vi "LJM read config.vi"(0 "Working Directory":path, 5 "filename":string="ljstreamud.cfg") -> (1 "Data File Prefix":string="data", 2 "Scan Rate (Hz)":dbl=500.0 format="%.3f", 3 "Graph History":i32=1000 min=0, 4 "# Channels":i32=4, 6 "Disable Scaling":bool, 8 "Max File Size (Bytes)":i32=1048576, 9 "Write To File":bool, 10 "Channel Setup":T1={"+Ch"=["0", "1", "2", "3", "4", "5", "6", "7"], "-Ch"=["199", "199", "199", "199", "199", "199", "199", "199"], "Ranges"=[0, 0, 0, 0, 0, 0, 0, 0], "Scaling Equation"=["y=v0", "y=v1", "y=v2", "y=v3", "y=v4", "y=v5", "y=v6", "y=v7"], "Graph?"=[]} {"Ranges" items=["LJ_rgBIP10V", "LJ_rgBIP5V", "LJ_rgUNI5V", "LJ_rgUNI2P5V", "LJ_rgUNI1P25V", "LJ_rgBIP1V", "LJ_rgUNIP625V", "LJ_rgBIPP1V", "LJ_rgBIPP01V"]}, 11 "Good Experiment Config":bool, 12 "Interval (ms)":u32=500, 13 "Resolution":u8, 14 "SettlingFactor":u8, 15 "error out":errorcluster)   [LabVIEW 2025]
uses:
  <vilib>/Utility/config.llb/Read Key (String).vi
  <vilib>/Utility/config.llb/Read Key (U32).vi
  <vilib>/Utility/config.llb/Read Key (Double).vi
  <vilib>/Utility/config.llb/Read Key (I32).vi
  <vilib>/Utility/config.llb/Read Key (Boolean).vi
  <vilib>/Utility/config.llb/NI_LVConfig.lvlib
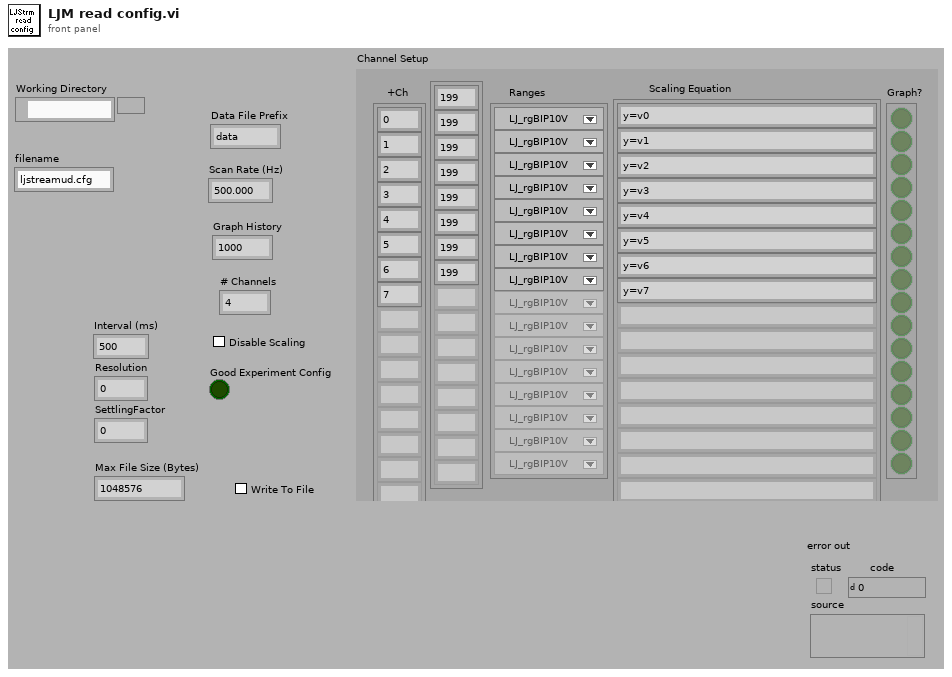
[diagram p1: front panel]
types:
  T1 = cluster{"+Ch":string[], "-Ch":string[], "Ranges":u16[], "Scaling Equation":string[], "Graph?":bool[]}
  T2 = typedef "NI_LVConfig.lvlib/Config Data RefNum.ctl" = refnum<k1>
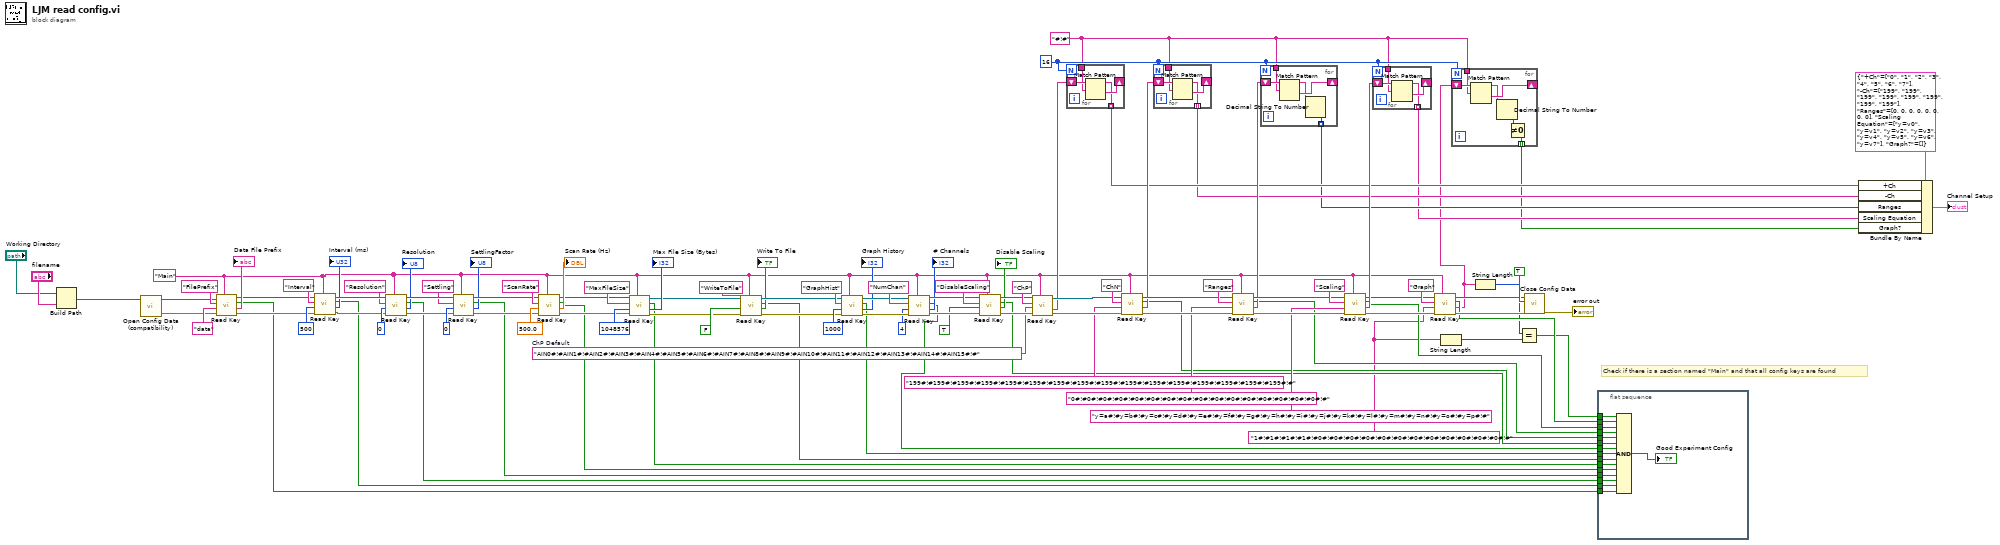
[diagram p0: block diagram]
diagram:
  w1 = "AIN0#!#AIN1#!#AIN2#!#AIN3#!#AIN4#!#AIN5#!#AIN6#!#AIN7#!#AIN8#!#AIN9#!#AIN10#!#AIN11#!#AIN12#!#AIN13#!#AIN14#!#AIN15#!#"  # ChP Default
  w5 = "1#!#1#!#1#!#1#!#0#!#0#!#0#!#0#!#0#!#0#!#0#!#0#!#0#!#0#!#0#!#0#!#" ("Data File Prefix")
  w69 = 16
  w68 = "#!#" ("delimiter (Tab)")
  w23 = "Main" ("section")
  # "Check if there is a section named \"Main\" and that all config keys are found"
  n1 = Build Path(base path="Working Directory", name or relative path="filename") -> (appended path=w108:path)
  n2 = call <vilib>:"Open Config Data (compatibility).vi"("configuration file path"=w108) -> ("error out"=w7:errorcluster, "refnum"=w8:T2)  [unwired: 8 in, 1 out]
  n3 = call-poly <vilib>:"Read Key.vi"("section"=w23, "error in (no error)"=w7, "default value"="data" ("Data File Prefix"), "key"="FilePrefix", "refnum"=w8) -> ("error out"=w43:errorcluster, "value"=→"Data File Prefix":string, "found?"=w22:bool, "refnum out"=w41:T2)  [unwired: 3 in]
  n4 = call-poly <vilib>:"Read Key.vi"("section"=w23, "error in (no error)"=w43, "default value"=u32 500 ("Scan Rate (Hz)"), "key"="Interval", "refnum"=w41) -> ("error out"=w48:errorcluster, "value"=→"Interval (ms)":u32, "found?"=w21:bool, "refnum out"=w47:T2)  [unwired: 3 in]
  n5 = call-poly <vilib>:"Read Key.vi"("section"=w23, "error in (no error)"=w48, "default value"=u8 0 ("Graph History"), "key"="Resolution", "refnum"=w47) -> ("error out"=w50:errorcluster, "value"=→"Resolution":u32, "found?"=w20:bool, "refnum out"=w49:T2)  [unwired: 3 in]
  n6 = call-poly <vilib>:"Read Key.vi"("section"=w23, "error in (no error)"=w50, "default value"=u8 0 ("# Channels"), "key"="Settling", "refnum"=w49) -> ("error out"=w42:errorcluster, "value"=→"SettlingFactor":u32, "found?"=w19:bool, "refnum out"=w40:T2)  [unwired: 3 in]
  n7 = call-poly <vilib>:"Read Key.vi"("section"=w23, "error in (no error)"=w42, "default value"=500.0 ("Scan Rate (Hz)"), "key"="ScanRate", "refnum"=w40) -> ("error out"=w33:errorcluster, "value"=→"Scan Rate (Hz)":dbl, "found?"=w18:bool, "refnum out"=w32:T2)  [unwired: 3 in]
  n8 = call-poly <vilib>:"Read Key.vi"("section"=w23, "error in (no error)"=w33, "default value"=1048576 ("Graph History"), "key"="MaxFileSize", "refnum"=w32) -> ("error out"=w27:errorcluster, "value"=→"Max File Size (Bytes)":i32, "found?"=w17:bool, "refnum out"=w28:T2)  [unwired: 3 in]
  n9 = call-poly <vilib>:"Read Key.vi"("section"=w23, "error in (no error)"=w27, "default value"=FALSE, "key"="WriteToFile", "refnum"=w28) -> ("error out"=w25:errorcluster, "value"=→"Write To File":bool, "found?"=w16:bool, "refnum out"=w26:T2)  [unwired: 3 in]
  n10 = call-poly <vilib>:"Read Key.vi"("section"=w23, "error in (no error)"=w25, "default value"=1000 ("Graph History"), "key"="GraphHist", "refnum"=w26) -> ("error out"=w102:errorcluster, "value"=→"Graph History":i32, "found?"=w15:bool, "refnum out"=w103:T2)  [unwired: 3 in]
  n11 = call-poly <vilib>:"Read Key.vi"("section"=w23, "error in (no error)"=w102, "default value"=4 ("# Channels"), "key"="NumChan", "refnum"=w103) -> ("error out"=w77:errorcluster, "value"=→"# Channels":i32, "found?"=w14:bool, "refnum out"=w78:T2)  [unwired: 3 in]
  n12 = call-poly <vilib>:"Read Key.vi"("section"=w23, "error in (no error)"=w77, "default value"=TRUE, "key"="DisableScaling", "refnum"=w78) -> ("error out"=w75:errorcluster, "value"=→"Disable Scaling":bool, "found?"=w13:bool, "refnum out"=w74:T2)  [unwired: 3 in]
  n13 = call-poly <vilib>:"Read Key.vi"("section"=w23, "error in (no error)"=w75, "default value"=w1, "key"="ChP", "refnum"=w74) -> ("error out"=w97:errorcluster, "value"=w83:string, "refnum out"=w98:T2)  [unwired: 3 in, 1 out]
  n14 = for {
    N: w69 -> [_]
    shift-right: [w111] -> _
    shift-left: w83 -> [w113]
    tunnel: w68 -> [w112]
    tunnel: [w110] -> w59 mode=indexing
    n15 = Match Pattern(string=w113, regular expression=w112) -> (before substring=w110:string, after substring=w111:string)  [unwired: 1 in, 2 out]
  }
  n16 = call-poly <vilib>:"Read Key.vi"("section"=w23, "error in (no error)"=w97, "default value"="199#!#199#!#199#!#199#!#199#!#199#!#199#!#199#!#199#!#199#!#199#!#199#!#199#!#199#!#199#!#199#!#" ("Data File Prefix"), "key"="ChN", "refnum"=w98) -> ("error out"=w96:errorcluster, "value"=w82:string, "found?"=w12:bool, "refnum out"=w95:T2)  [unwired: 3 in]
  n17 = for {
    N: w69 -> [_]
    shift-right: [w115] -> _
    shift-left: w82 -> [w117]
    tunnel: w68 -> [w116]
    tunnel: [w114] -> w58 mode=indexing
    n18 = Match Pattern(string=w117, regular expression=w116) -> (before substring=w114:string, after substring=w115:string)  [unwired: 1 in, 2 out]
  }
  n19 = call-poly <vilib>:"Read Key.vi"("section"=w23, "error in (no error)"=w96, "default value"="0#!#0#!#0#!#0#!#0#!#0#!#0#!#0#!#0#!#0#!#0#!#0#!#0#!#0#!#0#!#0#!#" ("Data File Prefix"), "key"="Ranges", "refnum"=w95) -> ("error out"=w93:errorcluster, "value"=w81:string, "found?"=w11:bool, "refnum out"=w92:T2)  [unwired: 3 in]
  n20 = for {
    N: w69 -> [_]
    shift-right: [w120] -> _
    shift-left: w81 -> [w122]
    tunnel: w68 -> [w121]
    tunnel: [w118] -> w57 mode=indexing
    n21 = Match Pattern(string=w122, regular expression=w121) -> (before substring=w119:string, after substring=w120:string)  [unwired: 1 in, 2 out]
    n22 = Decimal String To Number(string=w119) -> (number=w118:i32)  [unwired: 2 in, 1 out]
  }
  n23 = call-poly <vilib>:"Read Key.vi"("section"=w23, "error in (no error)"=w93, "default value"="y=a#!#y=b#!#y=c#!#y=d#!#y=e#!#y=f#!#y=g#!#y=h#!#y=i#!#y=j#!#y=k#!#y=l#!#y=m#!#y=n#!#y=o#!#y=p#!#" ("Data File Prefix"), "key"="Scaling", "refnum"=w92) -> ("error out"=w72:errorcluster, "value"=w80:string, "found?"=w10:bool, "refnum out"=w67:T2)  [unwired: 3 in]
  n24 = for {
    N: w69 -> [_]
    shift-right: [w124] -> _
    shift-left: w80 -> [w126]
    tunnel: w68 -> [w125]
    tunnel: [w123] -> w56 mode=indexing
    n25 = Match Pattern(string=w126, regular expression=w125) -> (before substring=w123:string, after substring=w124:string)  [unwired: 1 in, 2 out]
  }
  n26 = call-poly <vilib>:"Read Key.vi"("section"=w23, "error in (no error)"=w72, "default value"=w5, "key"="Graph", "refnum"=w67) -> ("error out"=w71:errorcluster, "value"=w6:string, "found?"=w9:bool, "refnum out"=w70:T2)  [unwired: 3 in]
  n27 = String Length(string=w5) -> (length=w3:i32)
  n28 = for {
    N: w69 -> [_]
    shift-right: [w130] -> _
    shift-left: w6 -> [w132]
    tunnel: w68 -> [w131]
    tunnel: [w127] -> w55 mode=indexing
    n29 = Match Pattern(string=w132, regular expression=w131) -> (before substring=w129:string, after substring=w130:string)  [unwired: 1 in, 2 out]
    n30 = Decimal String To Number(string=w129) -> (number=w128:i32)  [unwired: 2 in, 1 out]
    n31 = Not Equal To 0?(x=w128) -> (x != 0?=w127:bool)
  }
  n32 = String Length(string=w6) -> (length=w4:i32)
  n33 = Equal?(x=w4, y=w3) -> (x = y?=w2:bool)
  n34 = call <vilib>:"Close Config Data.vi"("error in (no error)"=w71, "write file if changed (T)"=TRUE ("write configuration file? (F)"), "refnum"=w70) -> ("error out"=→"error out":errorcluster)  [unwired: 7 in, 1 out]
  n35 = flat-sequence {
    tunnel: w22 -> [w148]
    tunnel: w21 -> [w147]
    tunnel: w20 -> [w146]
    tunnel: w19 -> [w145]
    tunnel: w18 -> [w144]
    tunnel: w17 -> [w143]
    tunnel: w16 -> [w142]
    tunnel: w15 -> [w141]
    tunnel: w14 -> [w140]
    tunnel: w13 -> [w139]
    tunnel: w12 -> [w138]
    tunnel: w11 -> [w137]
    tunnel: w10 -> [w136]
    tunnel: w9 -> [w135]
    tunnel: w2 -> [w133]
    frame #0 {
      n36 = Compound Arithmetic op=AND(w133, w135, w136, w137, w138, w139, w140, w141, w142, w143, w144, w145, w146, w147, w148) -> (→"Good Experiment Config":bool)
    }
  }
  n37 = Bundle By Name(cluster=T1 {"+Ch"=["0", "1", "2", "3", "4", "5", "6", "7"], "-Ch"=["199", "199", "199", "199", "199", "199", "199", "199"], "Ranges"=[0, 0, 0, 0, 0, 0, 0, 0], "Scaling Equation"=["y=v0", "y=v1", "y=v2", "y=v3", "y=v4", "y=v5", "y=v6", "y=v7"], "Graph?"=[]} ("Channel Setup"), "+Ch"=w59, "-Ch"=w58, "Ranges"=w57, "Scaling Equation"=w56, "Graph?"=w55) -> (→"Channel Setup":T1)
